vi "Autonomous Independent.vi"   [LabVIEW 2016]
doc: "This VI is called when autonomous begins, and will automatically be terminated when autonomous ends. You can carry out timed or sensor driven robot movement independently without needing to return to the caller."
uses:
  <vilib>/Rock Robotics/Network Tables/NT Read String.vi
  <vilib>/Rock Robotics/WPI/Ultrasonic/WPI_SonarMB1010AnalogGetRange.vi
  <vilib>/Rock Robotics/WPI/Utilities/WPI_GetSetVariantRefNum.vi
  <vilib>/Rock Robotics/Network Tables/NT Read Number.vi
  <vilib>/Rock Robotics/Network Tables/NT Write Numeric Array.vi
  <vilib>/Rock Robotics/Network Tables/NT Read String Array.vi
  <vilib>/Rock Robotics/Network Tables/NT Read Numeric Array.vi
  <vilib>/Rock Robotics/WPI/Ultrasonic/WPI_SonarMB1010AnalogRefNum Registry Get.vi
panel:
  # "Be sure to right-click and choose Data Operations>>Make Current Value default if you want to save the array values with the VI"
types:
  T1 = typedef "WPI_JoystickDevRef.ctl" = cluster{"Device":T2}
  T2 = typedef "WPI_JoystickDeviceEnum.ctl" = enum16{"USB 0", "USB 1", "USB 2", "USB 3", "USB 4", "USB 5"}
  T3 = enum16{"Front Left", "Front Right", "Back Left", "Back Right"}
  T4 = cluster{"Yaw":dbl, "Roll":dbl, "Pitch":dbl, "Heading":dbl, "Fused Heading":dbl}
  T5 = typedef "WPI_SonarMB1010AnalogDeviceRef.ctl" = cluster{"AIDeviceRef":T6, "Scaling factor (V/in)":dbl, "Average Bits":u8}
  T6 = typedef "WPI_AnalogChannelDevRef.ctl" = cluster{"DevStatus":errorcluster, "Analog Channel":T7}
  T7 = typedef "FPGA_AIChannel.ctl" = enum8{"AI 0", "AI 1", "AI 2", "AI 3", "AI MXP 0", "AI MXP 1", "AI MXP 2", "AI MXP 3", "Invalid"}
  T8 = typedef "WPI_MotorControlDeviceRef.ctl" = cluster{"DeviceStatus":errorcluster, "Type":T9, "PWM":cluster{"PWM Channel":T10, "DeadBand":T11}, "CAN":cluster{"Device Number":u8, "SetOutput VI Ref":variant, "GetOutput VI Ref":variant, "Enable VI Ref":variant, "Disable VI Ref":variant, "Data":variant}, "Invert":bool}
  T9 = typedef "WPI_MotorControlType.ctl" = enum16{"PWM", "CAN"}
  T10 = typedef "FPGA_DIOPWMChannel.ctl" = enum8{"PWM 0", "PWM 1", "PWM 2", "PWM 3", "PWM 4", "PWM 5", "PWM 6", "PWM 7", "PWM 8", "PWM 9", "PWM MXP 0", "PWM MXP 1", "PWM MXP 2", "PWM MXP 3", "PWM MXP 4", "PWM MXP 5", "PWM MXP 6", "PWM MXP 7", "PWM MXP 8", "PWM MXP 9", "Invalid"}
  T11 = typedef "WPI_PWMDeadband.ctl" = cluster{"Name":string, "maxPositivePwm":i32, "minPositivePwm":i32, "centerPwm":i32, "maxNegativePwm":i32, "minNegativePwm":i32, "angularRange":u16}
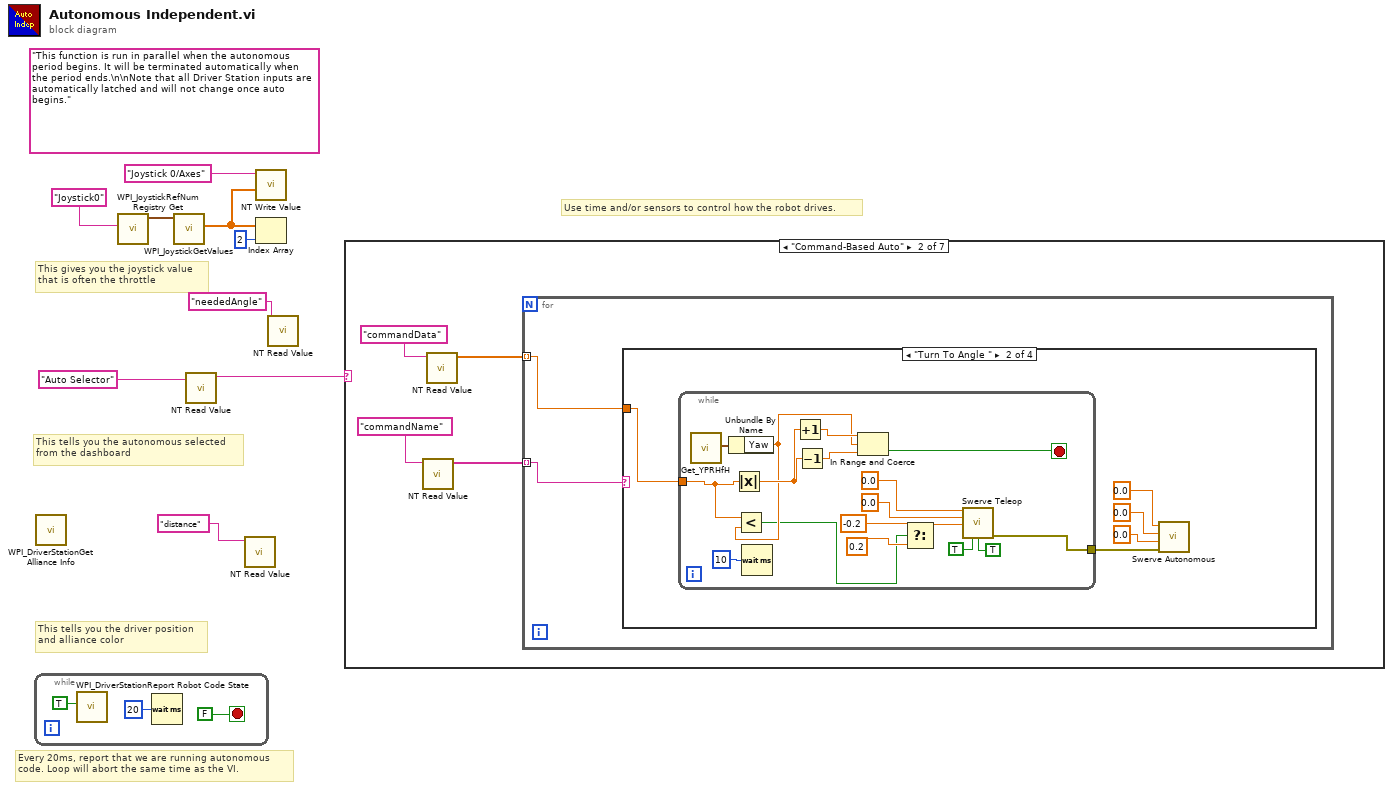
[diagram p0: block diagram]
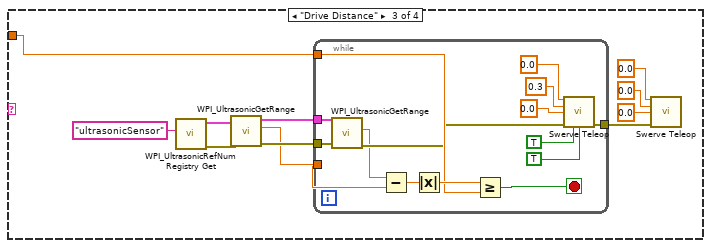
[diagram p4: hidden frame]
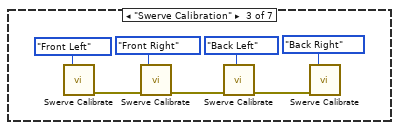
[diagram p6: hidden frame]
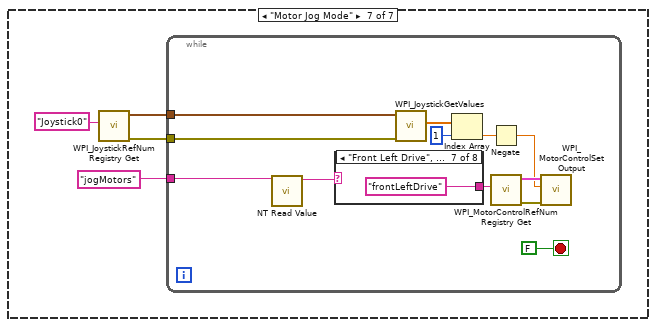
[diagram p10: hidden frame]
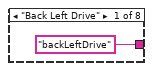
[diagram p11: hidden frame]
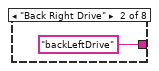
[diagram p12: hidden frame]
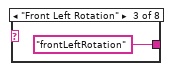
[diagram p13: hidden frame]
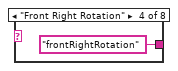
[diagram p14: hidden frame]
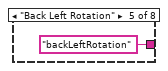
[diagram p15: hidden frame]
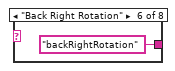
[diagram p16: hidden frame]
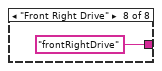
[diagram p17: hidden frame]
diagram:
  (unwired) "This function is run in parallel when the autonomous period begins. It will be terminated automatically when the period ends.\n\nNote that all Driver Station inputs are automatically latched and will not change once auto begins."
  # "This tells you the autonomous selected\nfrom the dashboard"
  # "Every 20ms, report that we are running autonomous\ncode. Loop will abort the same time as the VI."
  # "This gives you the joystick value\nthat is often the throttle"
  # "Use time and/or sensors to control how the robot drives."
  # "This tells you the driver position\nand alliance color"
  n1 = while {
    stop <- FALSE stop-if-true
    n2 = call <vilib>:"WPI_DriverStationReport Robot Code State.vi"("Autonomous"=TRUE) -> ()  [unwired: 10 in, 1 out]
    n3 = Wait (ms)(milliseconds to wait=u32 20) -> ()  [unwired: 1 out]
  }
  n4 = call <vilib>:"WPI_DriverStationGet Alliance Info.vi"() -> ()  [unwired: 12 out]
  n5 = call <vilib>:"WPI_JoystickRefNum Registry Get.vi"("refnum name"="Joystick0") -> ("JoystickDevRef"=w2:T1)  [unwired: 1 in, 9 out]
  n6 = call <vilib>:"WPI_JoystickGetValues.vi"("JoystickDevRef"=w2) -> ("Axes"=w4:dbl[])  [unwired: 6 in, 4 out]
  n7 = call-poly <vilib>:"NT Read Value.vi"("Name"="Auto Selector") -> ("String"=w8:string)  [unwired: 9 in, 1 out]
  n8 = call-poly <vilib>:"NT Read Value.vi"("Name"="distance") -> ()  [unwired: 9 in, 2 out]
  n9 = call-poly <vilib>:"NT Write Value.vi"("Numeric Array"=w4, "Name"="Joystick 0/Axes") -> ()  [unwired: 9 in, 1 out]
  n10 = Index Array(array=w4, index=2) -> ()  [unwired: 1 out]
  n11 = call-poly <vilib>:"NT Read Value.vi"("Name"="neededAngle") -> ()  [unwired: 9 in, 2 out]
  n12 = case shown="\"Command-Based Auto\"" w8 {
    frame Default {
      # "You can put your main auto here, or you can right-click on the case and make any\nother frame be the default case."
      # "This is the frame that will execute if no selection is made, or if it is not recognized"
    }
    frame "Command-Based Auto" {
      n13 = call-poly <vilib>:"NT Read Value.vi"("Name"="commandName") -> ("String Array"=w14:string[])  [unwired: 9 in, 1 out]
      n14 = call-poly <vilib>:"NT Read Value.vi"("Name"="commandData") -> ("Numeric Array"=w13:dbl[])  [unwired: 9 in, 1 out]
      n15 = for {
        tunnel: w14 -> [w18] mode=indexing
        tunnel: w13 -> [w17] mode=indexing
        n16 = case shown="\"Turn To Angle \"" w18 {
          tunnel: w17 -> [_ w19 w46 _]
          frame Default {
          }
          frame "Turn To Angle " {
            n17 = while {
              tunnel: [w38] -> w23
              tunnel: w19 -> [w26]
              stop <- w30 stop-if-true
              n18 = call <vilib>:"Get_YPRHfH.vi"() -> ("YRPHfH"=w39:T4)  [unwired: 11 in]
              n19 = Unbundle By Name(w39) -> ("Yaw"=w25:dbl)
              n20 = Absolute Value(x=w26) -> (abs(x)=w27:dbl)
              n21 = Less?(x=w26, y=w25) -> (x < y?=w24:bool)
              n22 = Wait (ms)(milliseconds to wait=u32 10) -> ()  [unwired: 1 out]
              n23 = Increment(x=w27) -> (x+1=w29:dbl)
              n24 = Decrement(x=w27) -> (x-1=w28:dbl)
              n25 = In Range and Coerce(upper limit=w29, x=w25, lower limit=w28) -> (In Range?=w30:bool)  [unwired: 1 out]
              n26 = Select(t=-0.2 ("Z"), s=w24, f=0.2 ("Z")) -> (s? t:f=w32:dbl)
              n27 = call "Swerve Teleop.vi"("X"=0.0, "Y"=0.0, "Z"=w32, "Robot Centric?"=TRUE, "Autonomous?"=TRUE ("Alternate Stop")) -> ("Error Out"=w38:errorcluster)  [unwired: 6 in, 4 out]
            }
            n28 = call "Swerve Autonomous.vi"("Error In"=w23, "Z"=0.0, "Y"=0.0, "X"=0.0) -> ()  [unwired: 7 in, 1 out]
          }
          frame "Drive Distance" {
            n29 = call-poly <vilib>:"WPI_UltrasonicRefNum Registry Get.vi"("refnum name"="ultrasonicSensor") -> ("error out"=w43:errorcluster, "SonarMB1010AnalogDevRef"=w45:T5)  [unwired: 9 in]
            n30 = call-poly <vilib>:"WPI_UltrasonicGetRange.vi"("error in"=w43, "SonarMB1010AnalogDevRef"=w45) -> ("error out"=w42:errorcluster, "Distance"=w41:dbl, "SonarMB1010AnalogDevRef"=w44:T5)  [unwired: 7 in]
            n31 = while {
              tunnel: [w59] -> w47
              tunnel: w41 -> [w58]
              tunnel: w46 -> [w56]
              tunnel: w44 -> [w55]
              tunnel: w42 -> [w54]
              stop <- w57 stop-if-true
              n32 = call-poly <vilib>:"WPI_UltrasonicGetRange.vi"("error in"=w54, "SonarMB1010AnalogDevRef"=w55) -> ("error out"=w53:errorcluster, "Distance"=w52:dbl)  [unwired: 7 in, 1 out]
              n33 = Subtract(x=w52, y=w58) -> (x-y=w66:dbl)
              n34 = Absolute Value(x=w66) -> (abs(x)=w65:dbl)
              n35 = Greater Or Equal?(x=w65, y=w56) -> (x >= y?=w57:bool)
              n36 = call "Swerve Teleop.vi"("X"=0.0, "Y"=0.3, "Z"=0.0, "Error In"=w53, "Robot Centric?"=TRUE, "Autonomous?"=TRUE) -> ("Error Out"=w59:errorcluster)  [unwired: 5 in, 4 out]
            }
            n37 = call "Swerve Teleop.vi"("X"=0.0, "Y"=0.0, "Z"=0.0, "Error In"=w47) -> ()  [unwired: 7 in, 5 out]
          }
          frame "Vision Align" {
          }
        }
      }
    }
    frame "Swerve Calibration" {
      n38 = call "Swerve Calibrate.vi"("Wheel Corner"=T3."Front Left") -> ("error out"=w69:errorcluster)  [unwired: 10 in]
      n39 = call "Swerve Calibrate.vi"("error in (no error)"=w69, "Wheel Corner"=T3."Front Right") -> ("error out"=w68:errorcluster)  [unwired: 9 in]
      n40 = call "Swerve Calibrate.vi"("error in (no error)"=w68, "Wheel Corner"=T3."Back Left") -> ("error out"=w67:errorcluster)  [unwired: 9 in]
      n41 = call "Swerve Calibrate.vi"("error in (no error)"=w67, "Wheel Corner"=T3."Back Right") -> ()  [unwired: 9 in, 1 out]
    }
    frame "Config 1" {
    }
    frame "Config 2" {
    }
    frame "Config 3" {
    }
    frame "Motor Jog Mode" {
      n42 = call <vilib>:"WPI_JoystickRefNum Registry Get.vi"("refnum name"="Joystick0") -> ("error out"=w76:errorcluster, "JoystickDevRef"=w77:T1)  [unwired: 1 in, 8 out]
      n43 = while {
        tunnel: w77 -> [w80]
        tunnel: w76 -> [w79]
        tunnel: "jogMotors" ("Name") -> [w78]
        stop <- FALSE stop-if-true
        n44 = call-poly <vilib>:"NT Read Value.vi"("Name"=w78) -> ("String"=w83:string)  [unwired: 9 in, 1 out]
        n45 = case shown="\"Front Left Drive\", Default" w83 {
          tunnel: ["backLeftDrive" ("refnum name") "backLeftDrive" ("refnum name") "frontLeftRotation" ("refnum name") "frontRightRotation" ("refnum name") "backLeftRotation" ("refnum name") "backRightRotation" ("refnum name") "frontLeftDrive" ("refnum name") "frontRightDrive" ("refnum name")] -> w82
          frame "Back Left Drive" {
          }
          frame "Back Right Drive" {
          }
          frame "Front Left Rotation" {
          }
          frame "Front Right Rotation" {
          }
          frame "Back Left Rotation" {
          }
          frame "Back Right Rotation" {
          }
          frame "Front Left Drive", Default {
          }
          frame "Front Right Drive" {
          }
        }
        n46 = call <vilib>:"WPI_JoystickGetValues.vi"("error in (no error)"=w79, "JoystickDevRef"=w80) -> ("Axes"=w89:dbl[])  [unwired: 5 in, 4 out]
        n47 = Index Array(array=w89, index=1) -> (element=w85:dbl)
        n48 = Negate(x=w85) -> (-x=w84:dbl)
        n49 = call <vilib>:"WPI_MotorControlRefNum Registry Get.vi"("refnum name"=w82) -> ("error out"=w87:errorcluster, "MotorControlDevRef"=w86:T8)  [unwired: 9 in]
        n50 = call <vilib>:"WPI_MotorControlSetOutput.vi"("error in (no error)"=w87, "Output"=w84, "MotorControlDevRef"=w86) -> ()  [unwired: 6 in, 3 out]
      }
    }
  }
